vi "init_singlepoint.vi"(7 "Analog_Input (in)":refnum<class "Analog_Input.lvclass">, 8 "error in":errorcluster, 9 "sample rate (Hz)":dbl=1.0, 10 "physical channels":tag="Dev3/ai0:2", 11 "samples per channel":i32=1000) -> (0 "error out":errorcluster, 3 "Analog_Input":refnum<class "Analog_Input.lvclass">)   [LabVIEW 2013, in "Analog_Input.lvclass"]
uses:
  Analog_Input.lvclass
  Experiment/Globals.vi
  <vilib>/DAQmx/create/channels.llb/DAQmx Create Channel (AI-Voltage-Basic).vi
  <vilib>/DAQmx/configure/timing.llb/DAQmx Timing (Sample Clock).vi
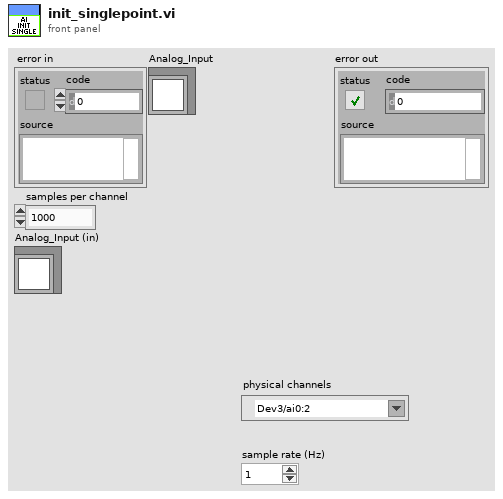
[diagram p1: front panel]
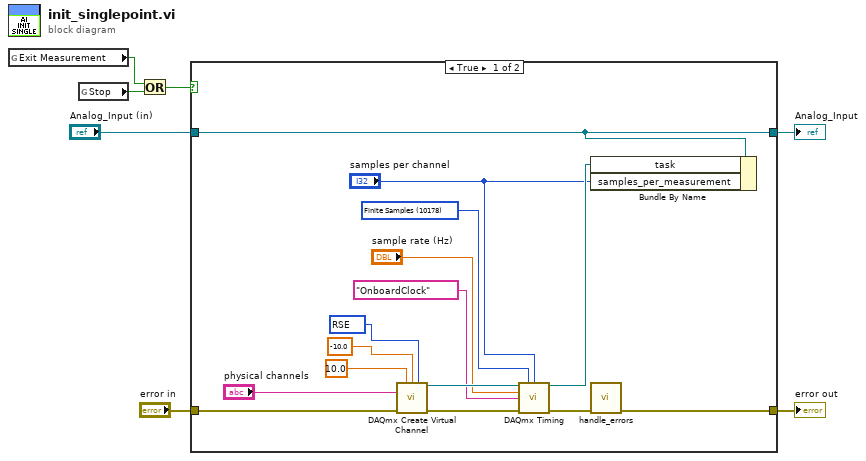
[diagram p0: block diagram]
diagram:
  n1 = global read "Globals.vi" "Exit Measurement"() -> (w3:bool)
  n2 = global read "Globals.vi" "Stop"() -> (w2:bool)
  n3 = Or(x=w3, y=w2) -> (x .or. y?=w1:bool)
  n4 = case shown="True" w1 {
    tunnel: "error in" -> [w13 w24]
    tunnel: [w10 w24] -> w6
    tunnel: "Analog_Input (in)" -> [w9 w23]
    tunnel: [w9 w23] -> w4
    frame True {
      w18 = 10178 items=["Finite Samples"=10178, "Continuous Samples"=10123, "Hardware Timed Single Point"=12522] ("sample mode")
      w21 = 10083 items=["default"=-1, "RSE"=10083, "NRSE"=10078, "Differential"=10106, "Pseudodifferential"=12529] ("input terminal configuration")
      n5 = call-poly <vilib>:"DAQmx Create Virtual Channel.vi"("maximum value"=10.0, "minimum value"=-10.0, "input terminal configuration"=w21, "physical channels"="physical channels", "error in"=w13) -> ("task out"=w20:refnum<k21>, "error out"=w19:errorcluster)  [unwired: 9 in]
      n6 = call-poly <vilib>:"DAQmx Timing.vi"("task/channels in"=w20, "sample mode"=w18, "samples per channel"="samples per channel", "rate"="sample rate (Hz)", "source"=tag "OnboardClock", "error in"=w19) -> ("task out"=w11:refnum<k21>, "error out"=w12:errorcluster)  [unwired: 8 in]
      n7 = Bundle By Name(cluster=w9, "task"=w11, "samples_per_measurement"="samples per channel") -> ()  [unwired: 1 out]
      n8 = call "handle_errors.vi"("error in (no error)"=w12) -> ("error out"=w10:errorcluster)  [unwired: 14 in]
    }
    frame False {
    }
  }
  "error out" <- w6
  "Analog_Input" <- w4
